vi "READ - File.vi"(0 "reference in":refnum<class "TEXT.lvclass">, 5 "error in (no error)":errorcluster, 7 "TDMS Path - READ":path) -> (14 "reference out":refnum<class "TEXT.lvclass">, 19 "error out":errorcluster)   [LabVIEW 2020, in "TEXT.lvclass"]
uses:
  TEXT.lvclass
  API/GSwFormDSP_class/functions/Attribute List.ctl
  API/GSwFormDSP_class/GSwFormDSP.lvclass
  API/Generic Utilities_class/Generic Utilities.lvclass
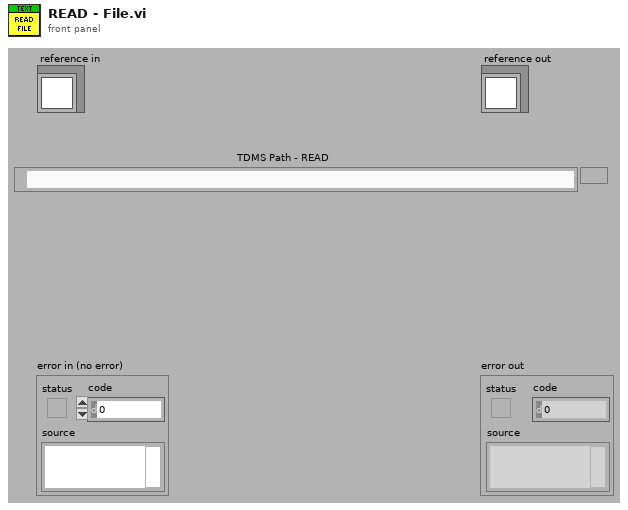
[diagram p1: front panel]
types:
  T1 = typedef "GSwFormDSP.lvclass/Attribute List.ctl" = string
  T2 = typedef "TEXT.lvclass/ObjectAttributesRef.ctl" = refnum<data-value>
  T3 = typedef "TEXT.lvclass/ObjectAttributes.ctl" = cluster{"Time Data":refnum<class "GSwFormDSP.lvclass">, "New Time Data Obj?":bool}
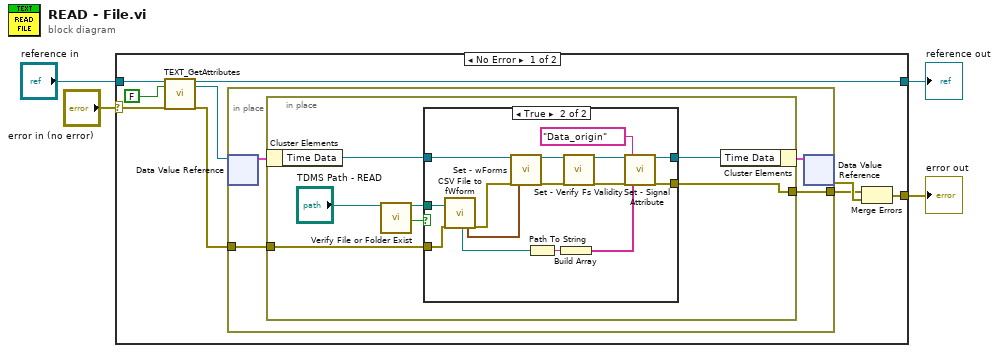
[diagram p0: block diagram]
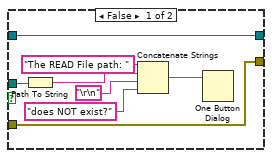
[diagram p2: hidden frame]
diagram:
  n1 = case shown="No Error" "error in (no error)" {
    selector: "error in (no error)" -> [w8 w49]
    tunnel: [w13 w49] -> w3
    tunnel: [w7 w48] -> w1
    tunnel: "reference in" -> [w10 w48]
    frame No Error {
      n2 = call "TEXT_GetAttributes.vi"("reference in"=w10, "return data? (T)"=FALSE, "error in (no error)"=w8) -> ("reference out"=w7:refnum<class "TEXT.lvclass">, "attributes ref"=w6:T2, "error out"=w5:errorcluster)  [unwired: 13 in, 1 out]
      n3 = in-place {
        in-place-border: [w14] -> w11
        in-place-border: w5 -> [w15]
        n4 = in-place-dvr #1(w6) -> (w16:T3)  [unwired: 1 out]
        n5 = in-place {
          in-place-border: w15 -> [w19]
          in-place-border: [w18] -> w14
          n6 = in-place-cluster #2(w16) -> ("Time Data"=w20:refnum<class "GSwFormDSP.lvclass">)
          n7 = call "Verify File or Folder Exist.vi"("path"="TDMS Path - READ") -> ("dup path"=w24:path, "file or folder exists?"=w23:bool)  [unwired: 16 in, 1 out]
          n8 = case shown="True" w23 {
            tunnel: w20 -> [w32 w47]
            tunnel: [w32 w45] -> w21
            tunnel: w24 -> [w30 w44]
            tunnel: w19 -> [w31 w43]
            tunnel: [w31 w46] -> w18
            frame False {
              n9 = Path To String(path=w30) -> (string=w28:string)
              n10 = Concatenate Strings("The READ File path: ", w28, "\r\n", "does NOT exist?") -> (w25:string)
              n11 = One Button Dialog(message=w25) -> ()  [unwired: 1 in, 1 out]
            }
            frame True {
              n12 = call "CSV File to fWform.vi"("CSV Path IN"=w44, "error in (no error)"=w43) -> ("CSV Path OUT"=w40:path, "wForms"=w41:waveform(dbl)[], "error out"=w42:errorcluster)  [unwired: 15 in]
              n13 = call "Set - wForms.vi"("reference in"=w47, "error in (no error)"=w42, "wForms"=w41) -> ("reference out"=w36:refnum<class "GSwFormDSP.lvclass">, "error out"=w34:errorcluster)  [unwired: 15 in]
              n14 = Path To String(path=w40) -> (string=w39:string)
              n15 = Build Array(w39) -> (w38:string[])
              n16 = call-dynamic "Set - Verify Fs Validity.vi"("reference in"=w36, "error in (no error)"=w34) -> ("reference in"=w35:refnum<class "GSwFormDSP.lvclass">, "error out"=w33:errorcluster)  [unwired: 16 in]
              n17 = call-dynamic "Set - Signal Attribute.vi"("reference in"=w35, "error in (no error)"=w33, "wForm Attributes"=T1 "Data_origin", "Attribute"=w38) -> ("reference in"=w45:refnum<class "GSwFormDSP.lvclass">, "error out"=w46:errorcluster)  [unwired: 14 in]
            }
          }
          n18 = in-place-cluster #2("Time Data"=w21) -> (w17:T3)
        }
        n19 = in-place-dvr #1(w17) -> (w12:errorcluster)  [unwired: 1 out]
      }
      n20 = Merge Errors(w11, w12) -> (w13:errorcluster)
    }
    frame Error {
    }
  }
  "error out" <- w3
  "reference out" <- w1
